vi "DigitalOut test-Modify.vi"() -> ()   [LabVIEW 2013]
panel:
  in  "PWM \nCounter-clockwise":dbl
  in  "PWM\nClockwise":dbl
  in  "STOP":bool
  # "DIGITALOUT Test"
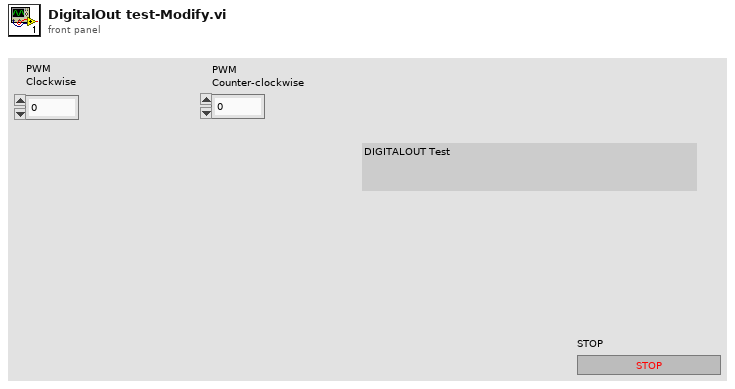
[diagram p1: front panel]
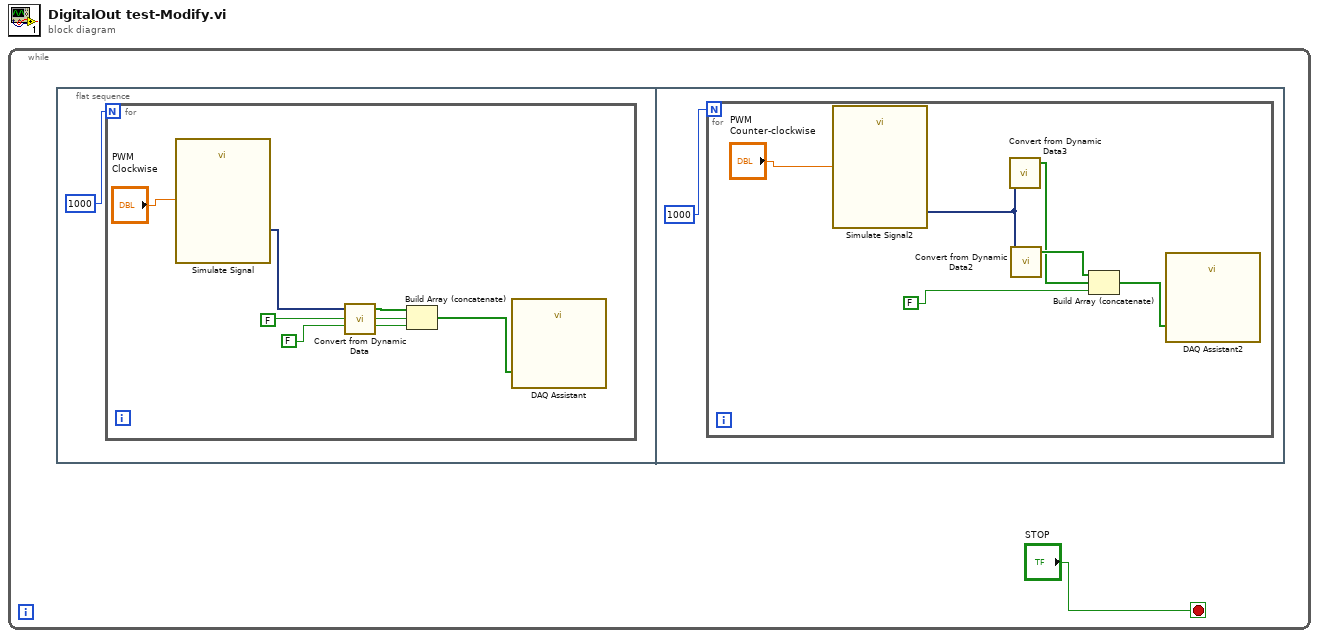
[diagram p0: block diagram]
diagram:
  n1 = while {
    stop <- "STOP" stop-if-true
    n2 = flat-sequence {
      frame #0 {
        n3 = for {
          N: 1000 -> [_]
          n4 = call "Simulate Signal"("Duty Cycle (%)"="PWM\nClockwise") -> ("Square"=w7:dynamicdata)  [unwired: 13 in, 1 out]
          n5 = call "Convert from Dynamic Data"("Dynamic Data Type"=w7) -> ("Array"=w6:bool[])  [unwired: 3 in]
          n6 = Build Array (concatenate)(w6, FALSE, FALSE) -> (w3:bool[])
          n7 = call "DAQ Assistant"("data"=w3) -> ()  [unwired: 17 in, 2 out]
        }
      }
      frame #1 {
        n8 = for {
          N: 1000 -> [_]
          n9 = call "Simulate Signal2"("Duty Cycle (%)"="PWM \nCounter-clockwise") -> ("Square"=w13:dynamicdata)  [unwired: 13 in, 1 out]
          n10 = call "Convert from Dynamic Data3"("Dynamic Data Type"=w13) -> ("Array"=w12:bool[])  [unwired: 3 in]
          n11 = call "Convert from Dynamic Data2"("Dynamic Data Type"=w13) -> ("Array"=w14:bool[])  [unwired: 3 in]
          n12 = Build Array (concatenate)(w14, w12, FALSE) -> (w10:bool[])
          n13 = call "DAQ Assistant2"("data"=w10) -> ()  [unwired: 17 in, 2 out]
        }
      }
    }
  }
